vi "Distance Test.vi"() -> ()   [LabVIEW 2017]
panel:
  in  "stop":bool
  in  "Inside?":bool
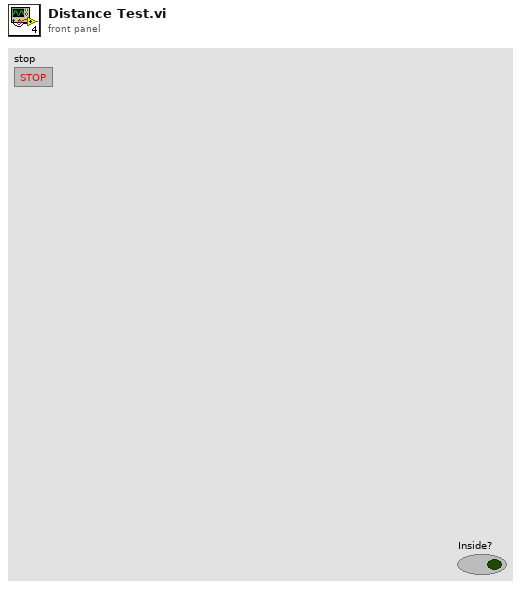
[diagram p1: front panel]
types:
  T1 = typedef "XY.ctl" = T2[]
  T2 = typedef "LidarPoint.ctl" = cluster{"X":dbl, "Y":dbl}
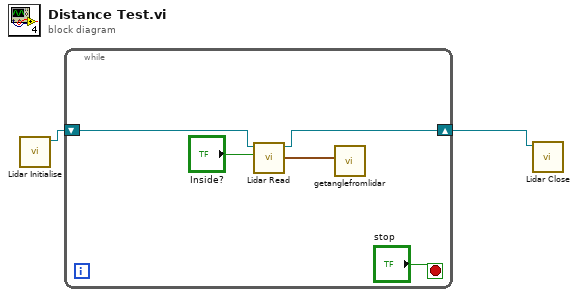
[diagram p0: block diagram]
diagram:
  n1 = call "Lidar Initialise.vi"() -> ("VISA resource name out"=w1:refnum<visa-resource-name>)  [unwired: 10 in, 1 out]
  n2 = while {
    shift-right: [w6] -> w2
    shift-left: w1 -> [w5]
    stop <- "stop" stop-if-true
    n3 = call "Lidar Read.vi"("Inside?"="Inside?", "VISA resource name"=w5) -> ("XY Array"=w4:T1, "VISA resource name out"=w6:refnum<visa-resource-name>)  [unwired: 4 in, 3 out]
    n4 = call "getanglefromlidar.vi"("XY Array"=w4) -> ()  [unwired: 5 in, 6 out]
  }
  n5 = call "Lidar Close.vi"("VISA resource name"=w2) -> ()  [unwired: 10 in, 1 out]
